vi "NET_Encoder_Values.vi"(8 "Read(F) Write(T)":bool, 11 "Encoder Counts":T1) -> (3 "Encoder Counts Out":T1)   [LabVIEW 2017]
uses:
  <vilib>/Rock Robotics/Network Tables/NT Read Numeric Array.vi
  <vilib>/Rock Robotics/Network Tables/NT Write Numeric Array.vi
  TypeDef/Cluster_Encoder_Count.ctl
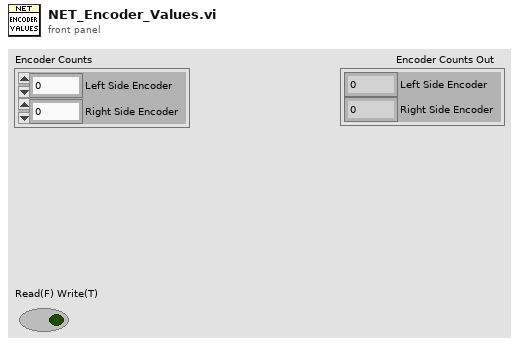
[diagram p1: front panel]
types:
  T1 = typedef "Cluster_Encoder_Count.ctl" = cluster{"Left Side Encoder":dbl, "Right Side Encoder":dbl}
  T2 = cluster{"Numeric Array[0]":dbl, "Numeric Array[1]":dbl}
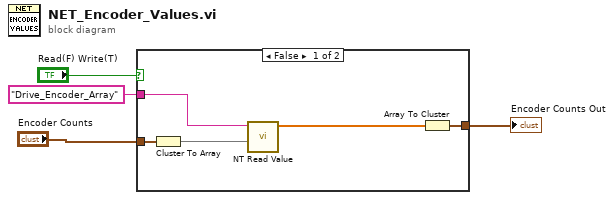
[diagram p0: block diagram]
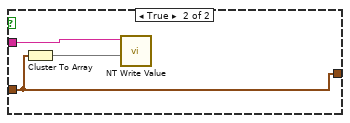
[diagram p2: hidden frame]
diagram:
  n1 = case shown="False" "Read(F) Write(T)" {
    tunnel: "Encoder Counts" -> [w8 w10]
    tunnel: "Drive_Encoder_Array" ("Name") -> [w9 w11]
    tunnel: [w5 w10] -> w2
    frame False {
      n2 = Cluster To Array(cluster=w8) -> (array=w7:dbl[])
      n3 = call-poly <vilib>:"NT Read Value.vi"("Default Value"=w7, "Name"=w9) -> ("Numeric Array"=w6:dbl[])  [unwired: 8 in, 1 out]
      n4 = Array To Cluster(array=w6) -> (cluster=w5:T2)
    }
    frame True {
      n5 = Cluster To Array(cluster=w10) -> (array=w12:dbl[])
      n6 = call-poly <vilib>:"NT Write Value.vi"("Numeric Array"=w12, "Name"=w11) -> ()  [unwired: 9 in, 1 out]
    }
  }
  "Encoder Counts Out" <- w2
